vi "PIEnable.vi"(8 "error in (no error)":errorcluster, 10 "Enable?":bool, 11 "connection ID":refnum<k16>) -> (0 "error out":errorcluster, 2 "Enable":bool, 3 "connection ID out":refnum<k16>)   [LabVIEW 2018]
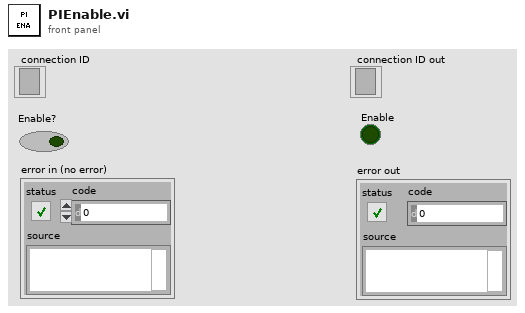
[diagram p1: front panel]
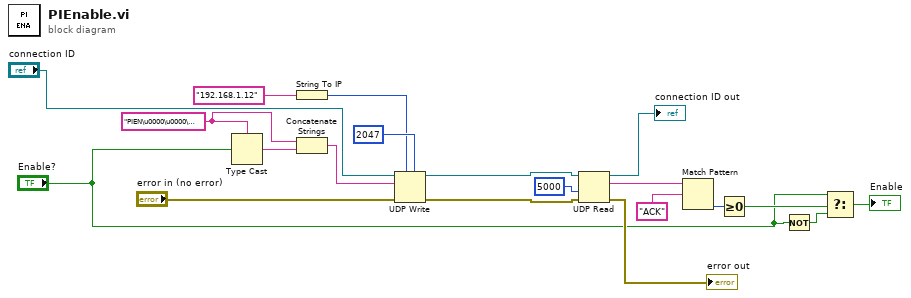
[diagram p0: block diagram]
diagram:
  w17 = "PIEN\u0000\u0000\u0000" ("data in")
  n1 = Type Cast(type=w17, x="Enable?") -> (*(type *) &x=w16:string)
  n2 = String To IP(1:"192.168.1.12" ("name")) -> (0:w13:u32)
  n3 = Concatenate Strings(w17, w16) -> (w18:string)
  n4 = UDP Write(address=w13, port or service name=u16 2047, connection ID="connection ID", data in=w18, 8:"error in (no error)") -> (error out=w20:errorcluster, 3:w19:refnum<k16>)  [unwired: 1 in]
  n5 = UDP Read(connection ID=w19, timeout ms (25000)=5000, 8:w20) -> (data out=w7:string, error out=→"error out":errorcluster, 3:→"connection ID out":refnum<k16>)  [unwired: 1 in, 2 out]
  n6 = Match Pattern(string=w7, regular expression="ACK" ("y")) -> (offset past match=w5:i32)  [unwired: 1 in, 3 out]
  n7 = Greater Or Equal To 0?(x=w5) -> (x >= 0?=w4:bool)
  n8 = Not(x="Enable?") -> (.not. x?=w2:bool)
  n9 = Select(t="Enable?", s=w4, f=w2) -> (s? t:f=→"Enable":bool)
